vi "Auto Nastawy.vi"(5 "queue":refnum<queue>, 8 "CAN ramki in":T1 {"type" items=["CAN Data", "CAN Remote"]; "identifier" format="%.0x"}) -> ()   [LabVIEW 2015]
uses:
  PC/ramki konfiguracyjne.ctl
  CANFrameControl.ctl
  PC/QMH Fundamentals - Message Cluster.ctl
  Enum nastawy.ctl
panel:
  in  "TYL L":T2={"Prąd"=20.0, "Kp"=10.0, "Ki"=3.0, "OK Button"=FALSE, "ID CAN"=2, "IDD"=3, "Sat"=250} {"Ki" format="%.1f"; "Kp" format="%.1f"; "Prąd" format="%.1f"}
  in  "SRODEK L":T2={"Prąd"=20.0, "Kp"=10.0, "Ki"=3.0, "OK Button"=FALSE, "ID CAN"=2, "IDD"=4, "Sat"=250} {"Ki" format="%.1f"; "Kp" format="%.1f"; "Prąd" format="%.1f"}
  in  "PRZOD L":T2={"Prąd"=20.0, "Kp"=10.0, "Ki"=3.0, "OK Button"=FALSE, "ID CAN"=2, "IDD"=2, "Sat"=250} {"Ki" format="%.1f"; "Kp" format="%.1f"; "Prąd" format="%.1f"}
  in  "TYL P":T2={"Prąd"=20.0, "Kp"=10.0, "Ki"=0.0, "OK Button"=FALSE, "ID CAN"=1, "IDD"=3, "Sat"=250} {"Ki" format="%.1f"; "Kp" format="%.1f"; "Prąd" format="%.1f"}
  in  "SRODEK P":T2={"Prąd"=20.0, "Kp"=10.0, "Ki"=3.0000000000000013, "OK Button"=FALSE, "ID CAN"=1, "IDD"=4, "Sat"=250} {"Ki" format="%.1f"; "Kp" format="%.1f"; "Prąd" format="%.1f"}
  in  "PRZOD P":T2={"Prąd"=20.0, "Kp"=10.000000000000004, "Ki"=3.0, "OK Button"=FALSE, "ID CAN"=1, "IDD"=2, "Sat"=250} {"Ki" format="%.1f"; "Kp" format="%.1f"; "Prąd" format="%.1f"}
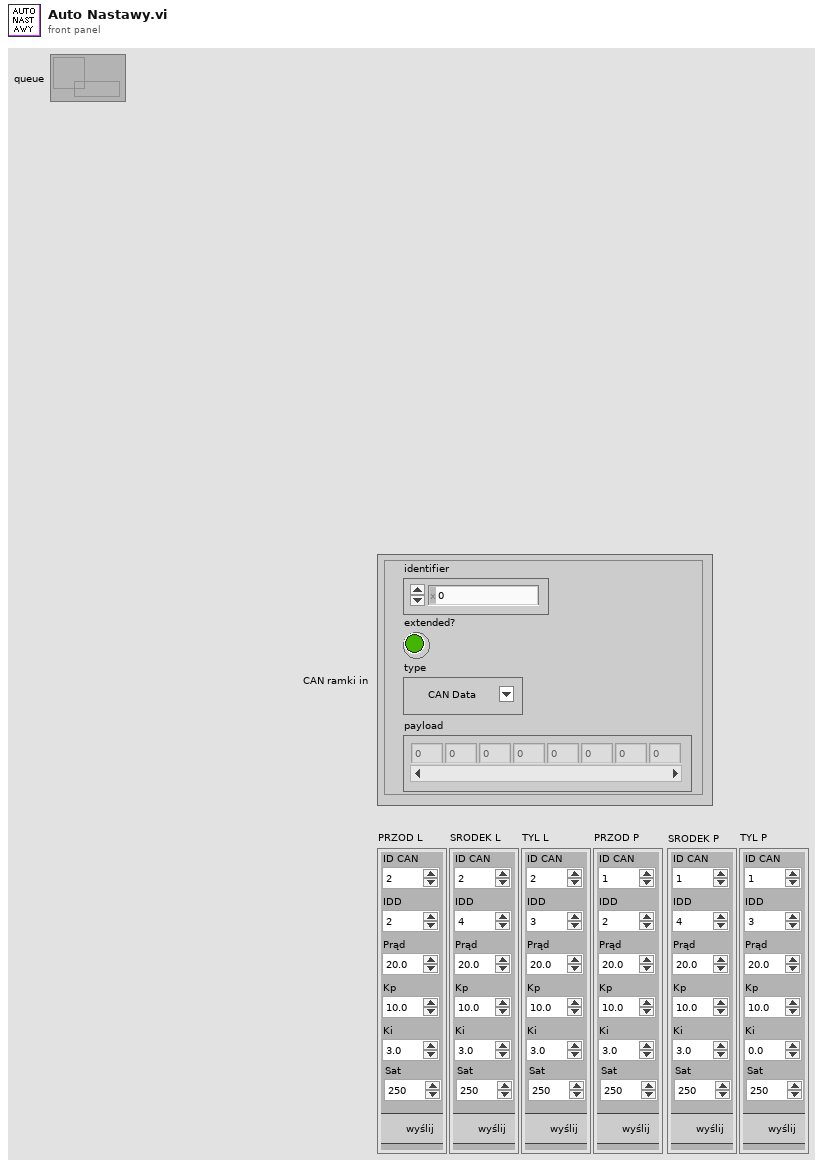
[diagram p1: front panel]
types:
  T1 = typedef "CANFrameControl.ctl" = cluster{"identifier":u32, "extended?":bool, "type":u8, "payload":u8[]}
  T2 = typedef "ramki konfiguracyjne.ctl" = cluster{"Prąd":dbl, "Kp":dbl, "Ki":dbl, "OK Button":bool, "ID CAN":u32, "IDD":u8, "Sat":u8}
  T3 = typedef "Enum nastawy.ctl" = enum16{"STOP", "PRZOD P", "SRODEK P", "TYL P", "PRZOD L", "SRODEK L", "TYL L"}
  T4 = typedef "QMH Fundamentals - Message Cluster.ctl" = cluster{"Message":string, "Message Data":variant}
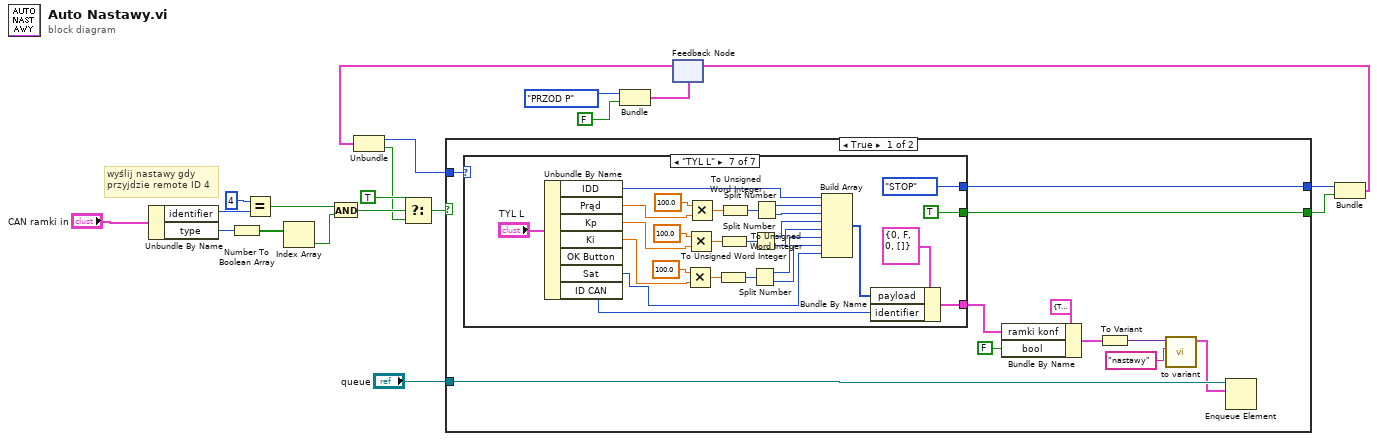
[diagram p0: block diagram]
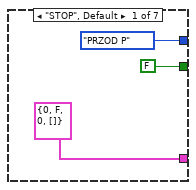
[diagram p2: hidden frame]
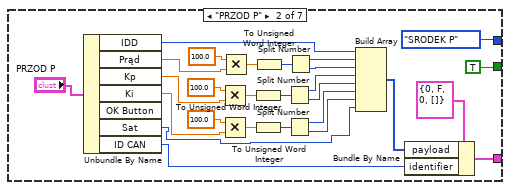
[diagram p3: hidden frame]
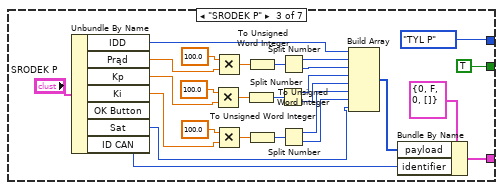
[diagram p4: hidden frame]
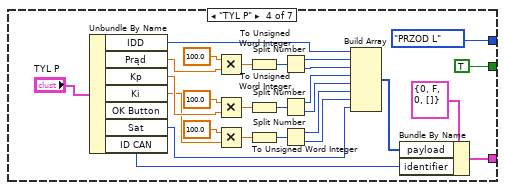
[diagram p5: hidden frame]
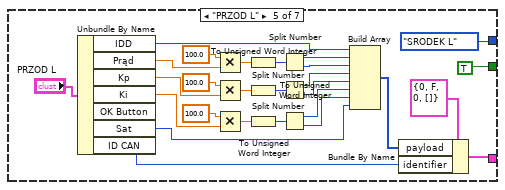
[diagram p6: hidden frame]
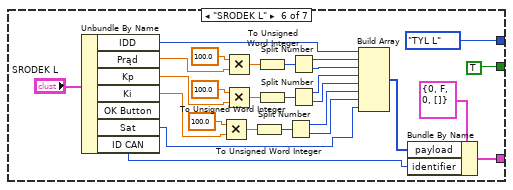
[diagram p7: hidden frame]
diagram:
  # "wyślij nastawy gdy \nprzyjdzie remote ID 4"
  n1 = Unbundle By Name("CAN ramki in") -> ("identifier"=w20:u32, "type"=w15:u8)
  n2 = Number To Boolean Array(number=w15) -> (Boolean array=w16:bool[])
  n3 = Equal?(x=u32 4, y=w20) -> (x = y?=w19:bool)
  n4 = Index Array(array=w16) -> (element=w17:bool)  [unwired: 1 in]
  n5 = And(x=w19, y=w17) -> (x .and. y?=w18:bool)
  n6 = Bundle(Enum_nastawy."PRZOD P", FALSE) -> (w4:cluster{T3, bool})  [unwired: 1 in]
  n7 = feedback #1(w4) -> (w2:cluster{T3, bool})
  n8 = Unbundle(w2) -> (w8:T3, w7:bool)
  n9 = Select(t=TRUE, s=w18, f=w7) -> (s? t:f=w12:bool)
  n10 = case shown="True" w12 {
    selector: w12 -> [_ w197]
    tunnel: w8 -> [w31 w198]
    tunnel: [w30 w198] -> w10
    tunnel: [w29 w197] -> w9
    tunnel: "queue" -> [w23 _]
    frame True {
      n11 = case shown="\"TYL L\"" w31 {
        tunnel: [T1 {"identifier"=0, "extended?"=FALSE, "type"=0, "payload"=[]} ("CAN frame 2") w44 w71 w98 w121 w152 w179] -> w22
        tunnel: [Enum_nastawy."PRZOD P" Enum_nastawy."SRODEK P" Enum_nastawy."TYL P" Enum_nastawy."PRZOD L" Enum_nastawy."SRODEK L" Enum_nastawy."TYL L" Enum_nastawy."STOP"] -> w30
        tunnel: [FALSE TRUE TRUE TRUE TRUE TRUE TRUE] -> w29
        frame "STOP", Default {
        }
        frame "PRZOD P" {
          n12 = Unbundle By Name("PRZOD P") -> ("IDD"=w43:u8, "Prąd"=w42:dbl, "Kp"=w41:dbl, "Ki"=w40:dbl, "Sat"=w35:u8, "ID CAN"=w36:u32)  [unwired: 1 out]
          n13 = Multiply(x=100.0, y=w41) -> (x*y=w52:dbl)
          n14 = Multiply(x=100.0, y=w40) -> (x*y=w47:dbl)
          n15 = Multiply(x=100.0, y=w42) -> (x*y=w57:dbl)
          n16 = To Unsigned Word Integer(number=w52) -> (unsigned 16bit integer=w54:u16)
          n17 = To Unsigned Word Integer(number=w47) -> (unsigned 16bit integer=w49:u16)
          n18 = To Unsigned Word Integer(number=w57) -> (unsigned 16bit integer=w60:u16)
          n19 = Split Number(x=w54) -> (hi(x)=w51:u8, lo(x)=w50:u8)
          n20 = Split Number(x=w49) -> (hi(x)=w46:u8, lo(x)=w45:u8)
          n21 = Split Number(x=w60) -> (hi(x)=w56:u8, lo(x)=w55:u8)
          n22 = Build Array(w43, w56, w55, w51, w50, w46, w45, w35) -> (w59:u8[])
          n23 = Bundle By Name(cluster=T1 {"identifier"=0, "extended?"=FALSE, "type"=0, "payload"=[]} ("CAN frame 2"), "payload"=w59, "identifier"=w36) -> (w44:T1)
        }
        frame "SRODEK P" {
          n24 = Unbundle By Name("SRODEK P") -> ("IDD"=w69:u8, "Prąd"=w68:dbl, "Kp"=w67:dbl, "Ki"=w66:dbl, "Sat"=w62:u8, "ID CAN"=w63:u32)  [unwired: 1 out]
          n25 = Multiply(x=100.0, y=w67) -> (x*y=w79:dbl)
          n26 = Multiply(x=100.0, y=w68) -> (x*y=w84:dbl)
          n27 = Multiply(x=100.0, y=w66) -> (x*y=w74:dbl)
          n28 = To Unsigned Word Integer(number=w79) -> (unsigned 16bit integer=w81:u16)
          n29 = To Unsigned Word Integer(number=w84) -> (unsigned 16bit integer=w87:u16)
          n30 = To Unsigned Word Integer(number=w74) -> (unsigned 16bit integer=w76:u16)
          n31 = Split Number(x=w81) -> (hi(x)=w78:u8, lo(x)=w77:u8)
          n32 = Split Number(x=w87) -> (hi(x)=w83:u8, lo(x)=w82:u8)
          n33 = Split Number(x=w76) -> (hi(x)=w73:u8, lo(x)=w72:u8)
          n34 = Build Array(w69, w83, w82, w78, w77, w73, w72, w62) -> (w86:u8[])
          n35 = Bundle By Name(cluster=T1 {"identifier"=0, "extended?"=FALSE, "type"=0, "payload"=[]} ("CAN frame 2"), "payload"=w86, "identifier"=w63) -> (w71:T1)
        }
        frame "TYL P" {
          n36 = Unbundle By Name("TYL P") -> ("IDD"=w97:u8, "Prąd"=w96:dbl, "Kp"=w95:dbl, "Ki"=w94:dbl, "Sat"=w90:u8, "ID CAN"=w89:u32)  [unwired: 1 out]
          n37 = Multiply(x=100.0, y=w96) -> (x*y=w111:dbl)
          n38 = Multiply(x=100.0, y=w95) -> (x*y=w106:dbl)
          n39 = Multiply(x=100.0, y=w94) -> (x*y=w101:dbl)
          n40 = To Unsigned Word Integer(number=w111) -> (unsigned 16bit integer=w114:u16)
          n41 = To Unsigned Word Integer(number=w106) -> (unsigned 16bit integer=w108:u16)
          n42 = To Unsigned Word Integer(number=w101) -> (unsigned 16bit integer=w103:u16)
          n43 = Split Number(x=w114) -> (hi(x)=w110:u8, lo(x)=w109:u8)
          n44 = Split Number(x=w108) -> (hi(x)=w105:u8, lo(x)=w104:u8)
          n45 = Split Number(x=w103) -> (hi(x)=w100:u8, lo(x)=w99:u8)
          n46 = Build Array(w97, w110, w109, w105, w104, w100, w99, w90) -> (w113:u8[])
          n47 = Bundle By Name(cluster=T1 {"identifier"=0, "extended?"=FALSE, "type"=0, "payload"=[]} ("CAN frame 2"), "payload"=w113, "identifier"=w89) -> (w98:T1)
        }
        frame "PRZOD L" {
          n48 = Unbundle By Name("PRZOD L") -> ("IDD"=w127:u8, "Prąd"=w128:dbl, "Kp"=w134:dbl, "Ki"=w140:dbl, "Sat"=w117:u8, "ID CAN"=w116:u32)  [unwired: 1 out]
          n49 = Multiply(x=100.0, y=w128) -> (x*y=w126:dbl)
          n50 = Multiply(x=100.0, y=w134) -> (x*y=w133:dbl)
          n51 = Multiply(x=100.0, y=w140) -> (x*y=w139:dbl)
          n52 = To Unsigned Word Integer(number=w126) -> (unsigned 16bit integer=w123:u16)
          n53 = To Unsigned Word Integer(number=w133) -> (unsigned 16bit integer=w131:u16)
          n54 = To Unsigned Word Integer(number=w139) -> (unsigned 16bit integer=w137:u16)
          n55 = Split Number(x=w123) -> (hi(x)=w129:u8, lo(x)=w130:u8)
          n56 = Split Number(x=w131) -> (hi(x)=w135:u8, lo(x)=w136:u8)
          n57 = Split Number(x=w137) -> (hi(x)=w141:u8, lo(x)=w142:u8)
          n58 = Build Array(w127, w129, w130, w135, w136, w141, w142, w117) -> (w124:u8[])
          n59 = Bundle By Name(cluster=T1 {"identifier"=0, "extended?"=FALSE, "type"=0, "payload"=[]} ("CAN frame 2"), "payload"=w124, "identifier"=w116) -> (w121:T1)
        }
        frame "SRODEK L" {
          n60 = Unbundle By Name("SRODEK L") -> ("IDD"=w150:u8, "Prąd"=w149:dbl, "Kp"=w148:dbl, "Ki"=w147:dbl, "Sat"=w144:u8, "ID CAN"=w143:u32)  [unwired: 1 out]
          n61 = Multiply(x=100.0, y=w147) -> (x*y=w155:dbl)
          n62 = Multiply(x=100.0, y=w149) -> (x*y=w165:dbl)
          n63 = Multiply(x=100.0, y=w148) -> (x*y=w160:dbl)
          n64 = To Unsigned Word Integer(number=w155) -> (unsigned 16bit integer=w157:u16)
          n65 = To Unsigned Word Integer(number=w165) -> (unsigned 16bit integer=w168:u16)
          n66 = To Unsigned Word Integer(number=w160) -> (unsigned 16bit integer=w162:u16)
          n67 = Split Number(x=w157) -> (hi(x)=w154:u8, lo(x)=w153:u8)
          n68 = Split Number(x=w168) -> (hi(x)=w164:u8, lo(x)=w163:u8)
          n69 = Split Number(x=w162) -> (hi(x)=w159:u8, lo(x)=w158:u8)
          n70 = Build Array(w150, w164, w163, w159, w158, w154, w153, w144) -> (w167:u8[])
          n71 = Bundle By Name(cluster=T1 {"identifier"=0, "extended?"=FALSE, "type"=0, "payload"=[]} ("CAN frame 2"), "payload"=w167, "identifier"=w143) -> (w152:T1)
        }
        frame "TYL L" {
          n72 = Unbundle By Name("TYL L") -> ("IDD"=w177:u8, "Prąd"=w176:dbl, "Kp"=w175:dbl, "Ki"=w174:dbl, "Sat"=w170:u8, "ID CAN"=w171:u32)  [unwired: 1 out]
          n73 = Multiply(x=100.0, y=w174) -> (x*y=w182:dbl)
          n74 = Multiply(x=100.0, y=w175) -> (x*y=w187:dbl)
          n75 = Multiply(x=100.0, y=w176) -> (x*y=w192:dbl)
          n76 = To Unsigned Word Integer(number=w182) -> (unsigned 16bit integer=w184:u16)
          n77 = To Unsigned Word Integer(number=w187) -> (unsigned 16bit integer=w189:u16)
          n78 = To Unsigned Word Integer(number=w192) -> (unsigned 16bit integer=w195:u16)
          n79 = Split Number(x=w184) -> (hi(x)=w181:u8, lo(x)=w180:u8)
          n80 = Split Number(x=w189) -> (hi(x)=w186:u8, lo(x)=w185:u8)
          n81 = Split Number(x=w195) -> (hi(x)=w191:u8, lo(x)=w190:u8)
          n82 = Build Array(w177, w191, w190, w186, w185, w181, w180, w170) -> (w194:u8[])
          n83 = Bundle By Name(cluster=T1 {"identifier"=0, "extended?"=FALSE, "type"=0, "payload"=[]} ("CAN frame 2"), "payload"=w194, "identifier"=w171) -> (w179:T1)
        }
      }
      n84 = Bundle By Name(cluster=cluster{"bool":bool, "ramki konf":T1} {"bool"=TRUE, "ramki konf"={"identifier"=0, "extended?"=TRUE, "type"=1, "payload"=[]}} ("jazda"), "ramki konf"=w22, "bool"=FALSE) -> (w24:cluster{"bool":bool, "ramki konf":T1})
      n85 = To Variant(anything=w24) -> (Variant=w27:variant)
      n86 = call "to variant.vi"("Message"="nastawy", "Variant"=w27) -> ("Message Cluster"=w21:T4)  [unwired: 9 in]
      n87 = Enqueue Element(queue=w23, element=w21) -> ()  [unwired: 2 in, 3 out]
    }
    frame False {
    }
  }
  n88 = Bundle(w10, w9) -> (w3:cluster{T3, bool})  [unwired: 1 in]
  n89 = feedback-in #1(w3) -> ()
